vi "Simple Capture Manager.vi"() -> ()   [LabVIEW 2016]
uses:
  Simple Capture Manager Controls/Simple Capture Notifier Type.ctl
  Simple Capture Manager Controls/Simple Capture Actions.ctl
  Hardware Configuration/Hardware Configuration Controls/Device Type.ctl
  Hardware Configuration/Hardware Configuration Controls/Device Function.ctl
  Device Library/Cameras/Ximea/Ximea Controls/Ximea Actions.ctl
  Device Library/Cameras/Ximea/Ximea Controls/Ximea Parameters.ctl
  Device Library/Cameras/Ximea/Ximea Controls/Ximea Parameter List.ctl
  Simple Capture Manager Controls/Simple Capture Scan Tracker.ctl
  Device Library/Lasers/Laser Controls/Laser Actions.ctl
  Device Library/Lasers/Laser Controls/Laser Settings.ctl
  Device Library/Lasers/Laser Controls/Laser Parameters.ctl
  Device Library/Stages/Stages Controls/Stage Actions.ctl
  Device Library/Cameras/Ximea/Ximea Controls/Ximea Notifier Element.ctl
  Device Library/Cameras/Ximea/Ximea Controls/Ximea ROI.ctl
  <vilib>/vision/Image Controls.llb/IMAQ Image.ctl
  Device Library/Cameras/Camera Controls/Camera IMAQ Key Info.ctl
  shell32.dll
panel:
  in  "Quit":bool
  in  "Main Tab":enum32{"Acquisition"}(tab)
  in  "Sampling Time (s)":dbl min=0.0 format="%#_2f"
  in  "Gain":dbl=0.1
  in  "Soft trigger":bool
  out "Current Cycle":u32
  out "Cycle":sgl(slide) scale=0.0..1.0
  in  "No. of Cycles":u32=1 min=1
  out "Frame":u32(slide) scale=0.0..40.0
  in  "Base Save Path":path
  in  "Capture":bool
  in  "Preview":bool
  out "Z Step":sgl(slide) scale=0.0..1.0
  in  "File Name":string="Test Image"
  in  "Exposure Time (s)":dbl=0.1
  in  "No. of Frames":u32=1 min=1
  in  "No. of Z Steps":u32=1 min=1
  in  "Z Step Size (µm)":dbl min=-10.0 max=10.0
  out "Current Step":u32
  out "Current Frame":u32
  in  "Subfolder Name":string="Area"
  # "Live Preview"
  # "Capture"
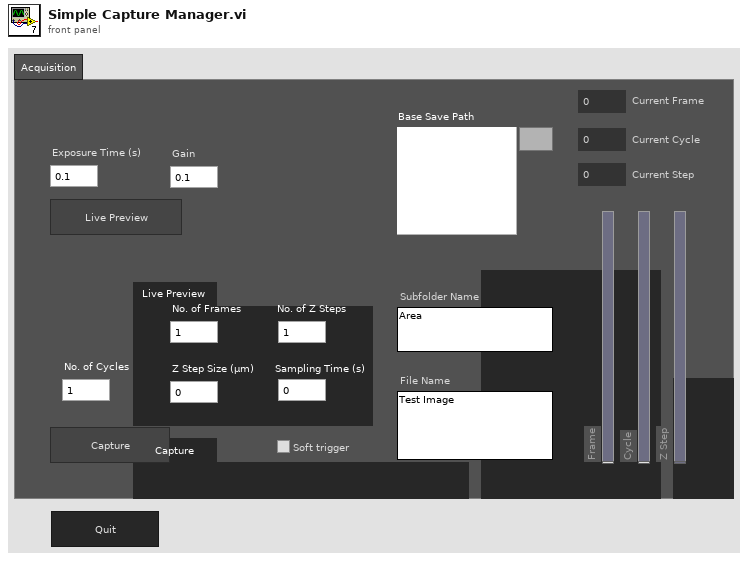
[diagram p1: front panel]
types:
  T1 = typedef "Simple Capture Notifier Type.ctl" = cluster{"No. of Frames ":u32, "No. of Z Steps":u32, "Z Step Size (µm)":dbl, "Exposure (s)":dbl, "Actions":T2, "No. of Cycles":u32, "Init Z Position (µm) ":dbl, "Base Path":path, "Save Path":path, "Metadata File Ref":refnum<file>, "Gain":dbl, "Running?":bool, "Sampling Time (s)":dbl}
  T2 = typedef "Simple Capture Actions.ctl" = enum16{"Preview", "Capture", "Laser On", "Laser Off", "Set Exposure/Gain", "Start Acquisition", "Update SubFolder", "Write Metadata", "Setup", "Camera", "Camera Soft Trigger", "Switch", "Cycle", "Step", "Abort", "Idle", "Quit"}
  T3 = typedef "Ximea Parameters.ctl" = cluster{"Parameter":T4, "Value":sgl}
  T4 = typedef "Ximea Parameter List.ctl" = enum16{"Exposure Time (s)", "Gain"}
  T5 = typedef "Device Function.ctl" = enum16{"Primary", "Secondary", "Overview", "Wide Field Drift Correction", "642 nm Excitation", "560 nm Excitation", "940 nm Excitation", "546 nm Excitation", "488 nm Excitation", "405 nm Excitation", "Objective Drift Correction", "4Pi Focus Lock", "4Pi Objective Lock", "Objective XY", "Objective Z", "Sample XY", "Sample Coarse Z", "Sample Z", "4Pi Lower", "4Pi Upper", "Mojo", "Adj Cavity", "Line Scanning", "Alert"}
  T6 = typedef "Device Type.ctl" = enum16{"AOTF", "Camera", "Deformable Mirror", "Laser", "Shutter", "Stage", "Waveform", "FPGA", "Email"}
  T7 = typedef "Ximea Actions.ctl" = enum16{"Idle", "Error Check", "Preview", "Record", "Soft Trigger", "Abort", "Record Settings", "Set Parameter", "Get Parameter", "Set ROI", "Get ROI", "Status", "Quit"}
  T8 = typedef "Simple Capture Scan Tracker.ctl" = cluster{"Current Step":u32, "Current Cycle":u32, "# of Cycles":u32, "# of Steps":u32}
  T9 = typedef "Laser Parameters.ctl" = enum16{"Wavelength (nm)", "Pulsing?", "Rep. Rate", "External Control", "Enable Fine", "Fine A", "Fine B", "Channel No."}
  T10 = typedef "Laser Settings.ctl" = cluster{"Laser Parameters":T9, "Value":dbl}
  T11 = typedef "Laser Actions.ctl" = enum16{"Error Check", "Set On/Off", "Set Power", "Set Parameter", "Get Power", "Get Status", "Get Parameter", "Quit"}
  T12 = typedef "Stage Actions.ctl" = enum16{"Get Position", "MVR", "MOVE", "HALT", "ONTARGET", "ERROR", "REFERENCE", "INIT", "VELOCITY", "STATUS", "EXIT", "HOME", "ZEROPOS", "NANOPOS", "ANALOG", "QUIT"}
  T13 = enum16{"open", "replace", "create", "open or create", "replace or create", "replace or create with confirmation"}
  T14 = typedef "Ximea Notifier Element.ctl" = cluster{"Ximea Actions":T7, "Received?":bool, "Ximea Parameter":T3, "Ximea ROI":T15, "Running?":bool, "File Path":path, "# of frames":u32, "Image Ref":T16, "Error":errorcluster, "Trigger?":bool, "ROI Increment":i32}
  T15 = typedef "Ximea ROI.ctl" = cluster{"H Offset":i32, "V Offset":i32, "H Width":i32, "V Width":i32}
  T16 = typedef "IMAQ Image.ctl" = refnum<image>
  T17 = typedef "Camera IMAQ Key Info.ctl" = cluster{"Frame":u32, "Sensor Height":i32, "Sensor Width":i32, "ROI Height":i32, "ROI Width":i32, "ROI Enable?":bool, "Bit per Pixel":u8}
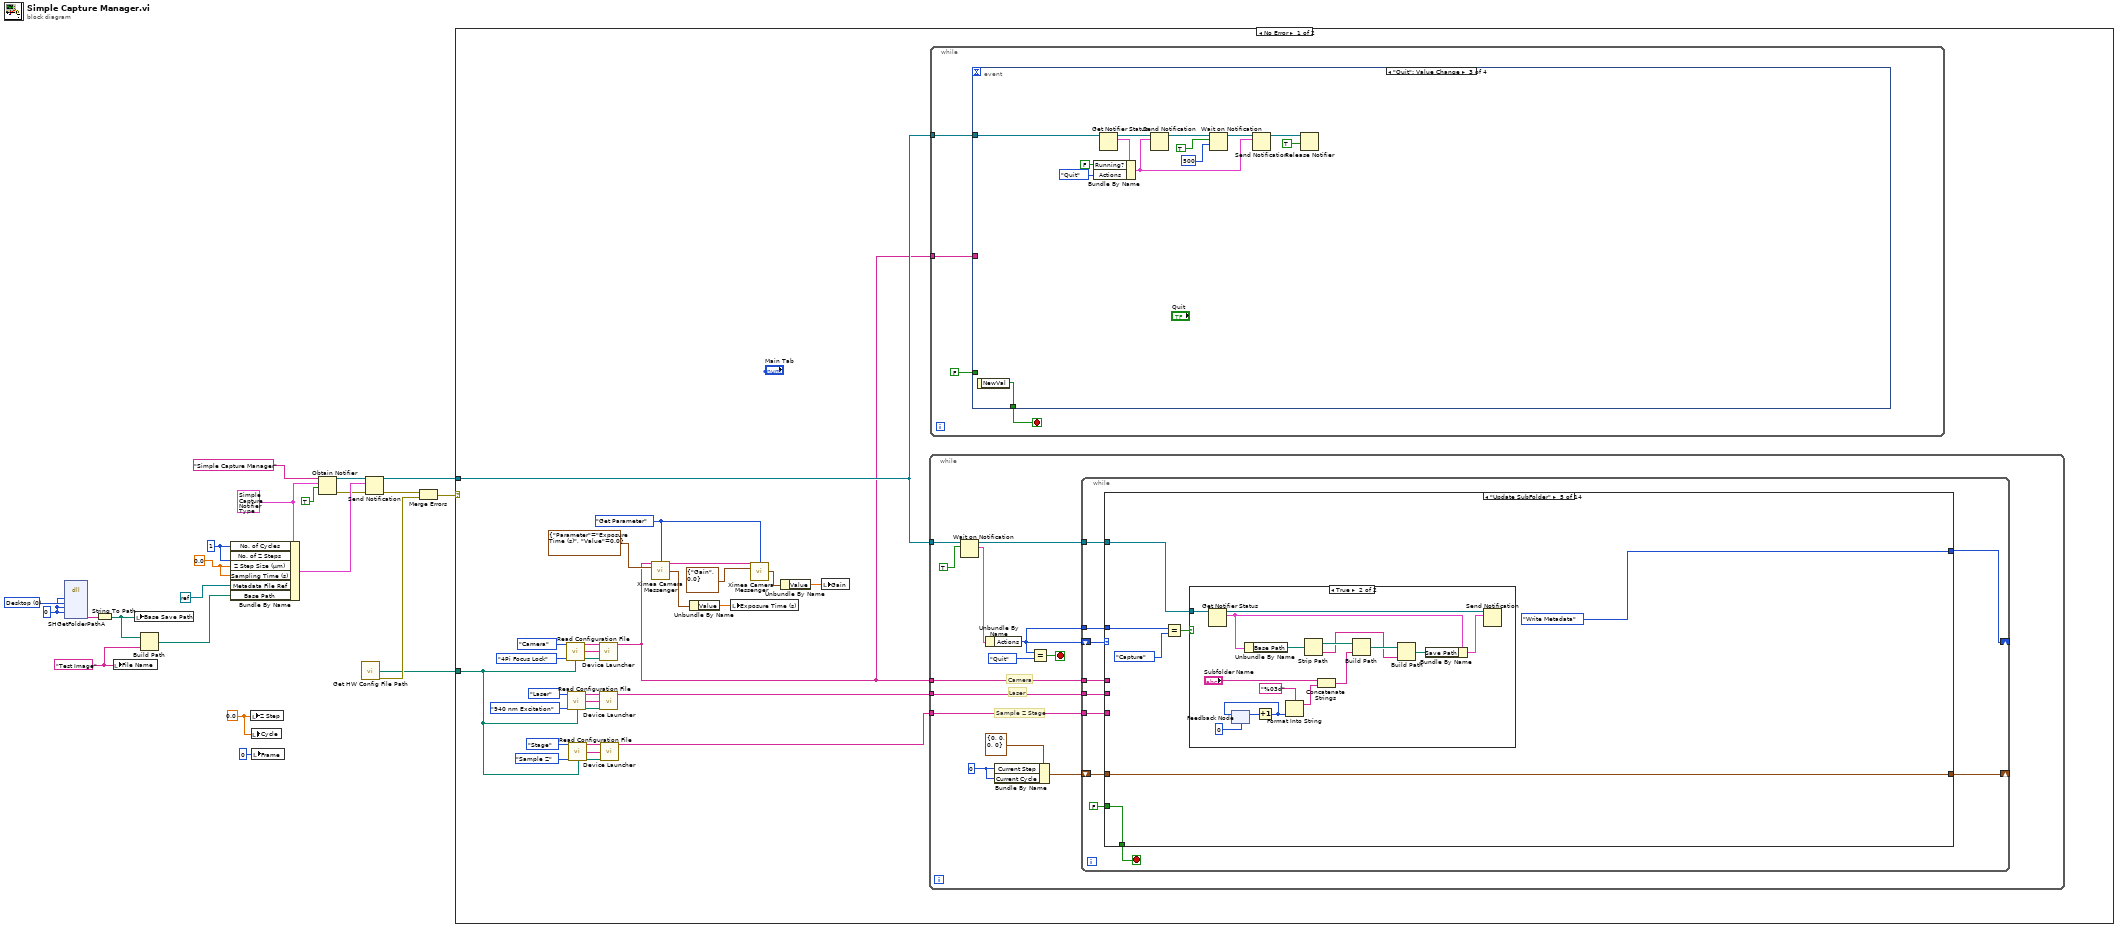
[diagram p0: block diagram]
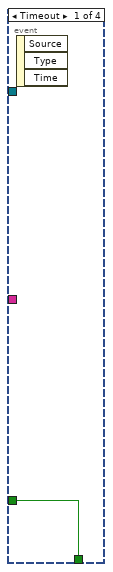
[diagram p2: hidden frame]
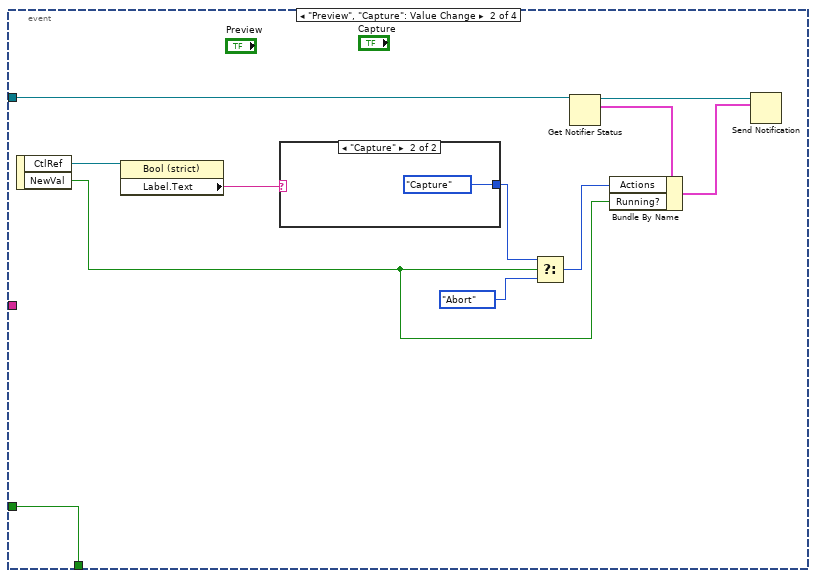
[diagram p3: hidden frame]
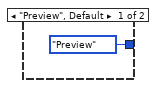
[diagram p4: hidden frame]
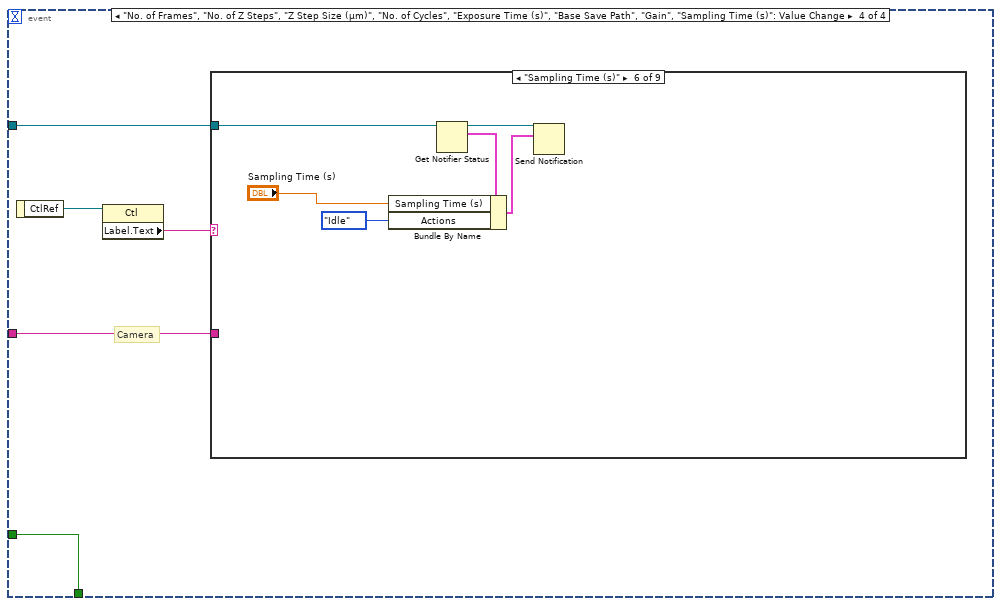
[diagram p5: hidden frame]
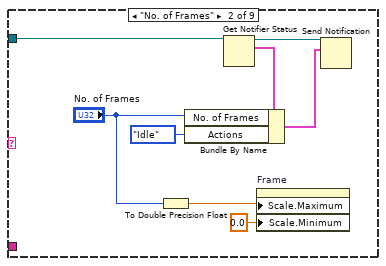
[diagram p7: hidden frame]
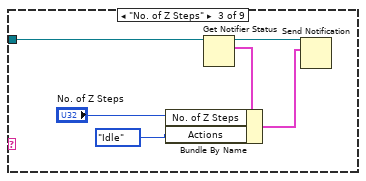
[diagram p8: hidden frame]
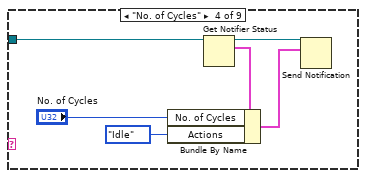
[diagram p9: hidden frame]
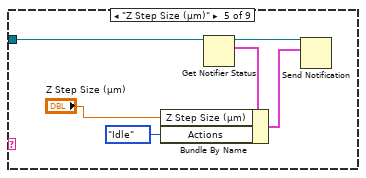
[diagram p10: hidden frame]
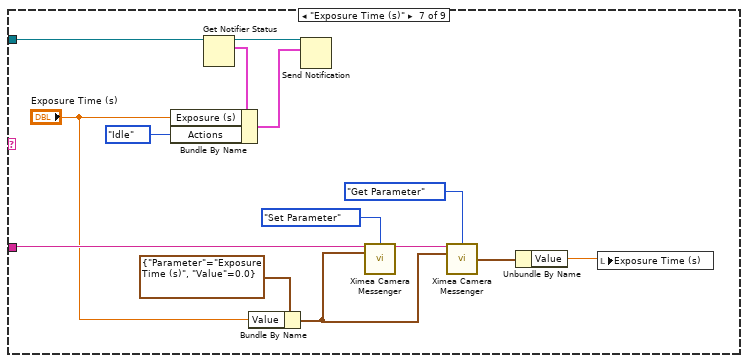
[diagram p11: hidden frame]
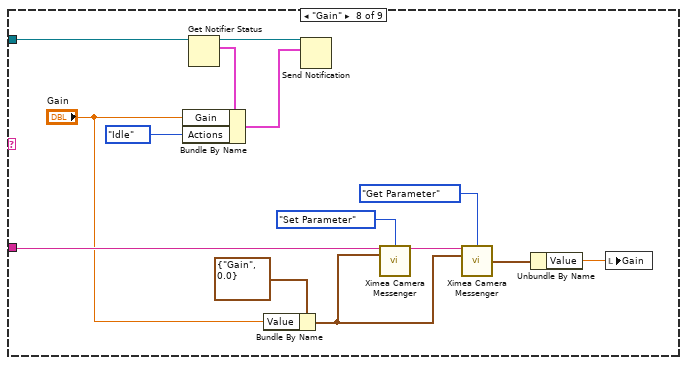
[diagram p12: hidden frame]
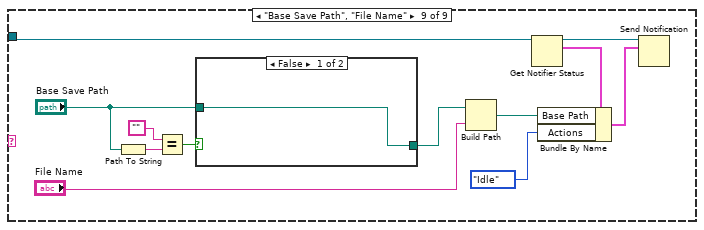
[diagram p13: hidden frame]
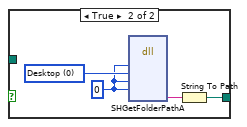
[diagram p14: hidden frame]
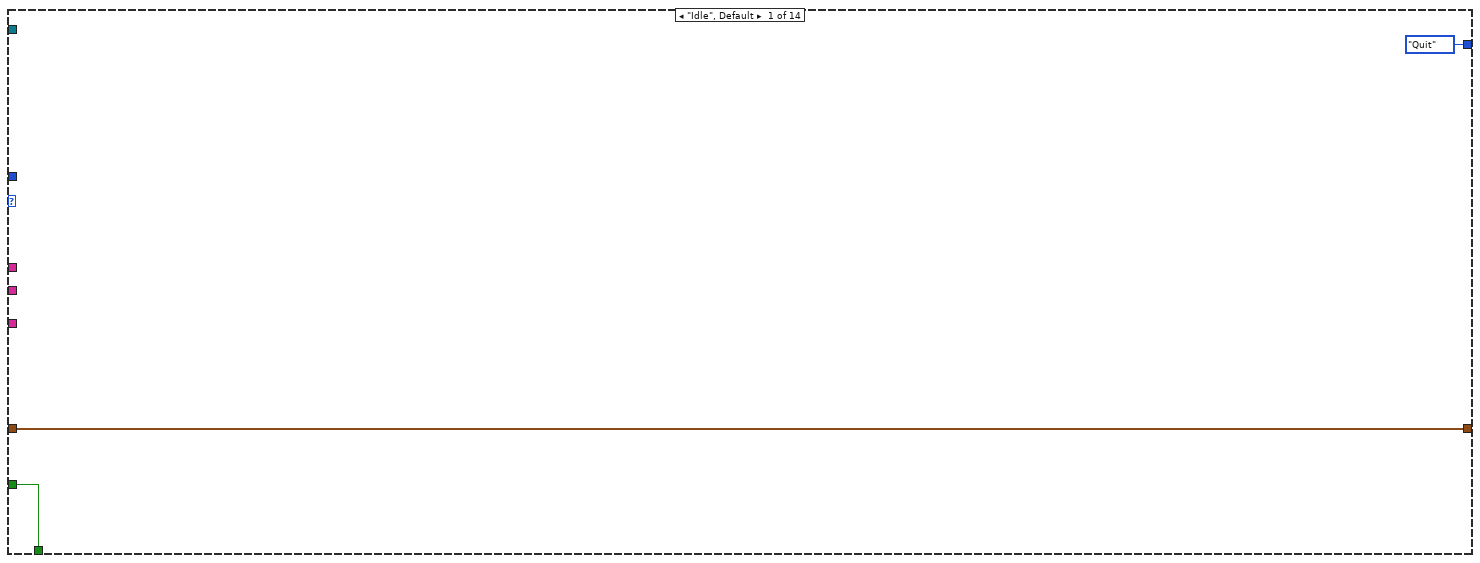
[diagram p15: hidden frame]
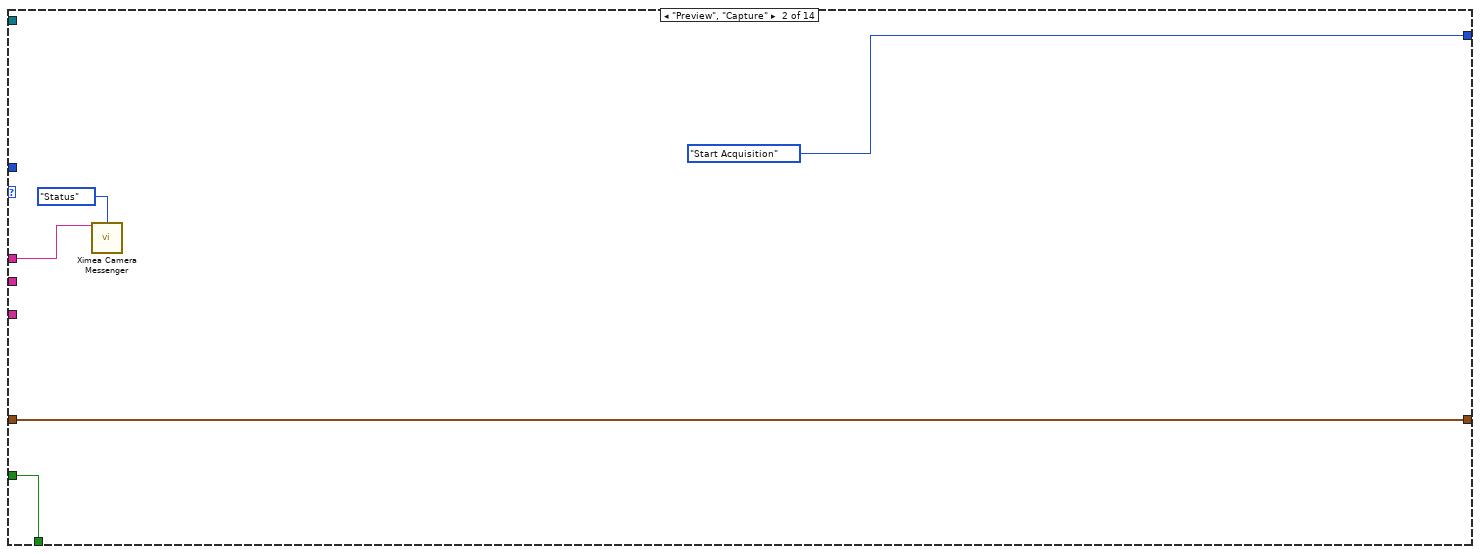
[diagram p16: hidden frame]
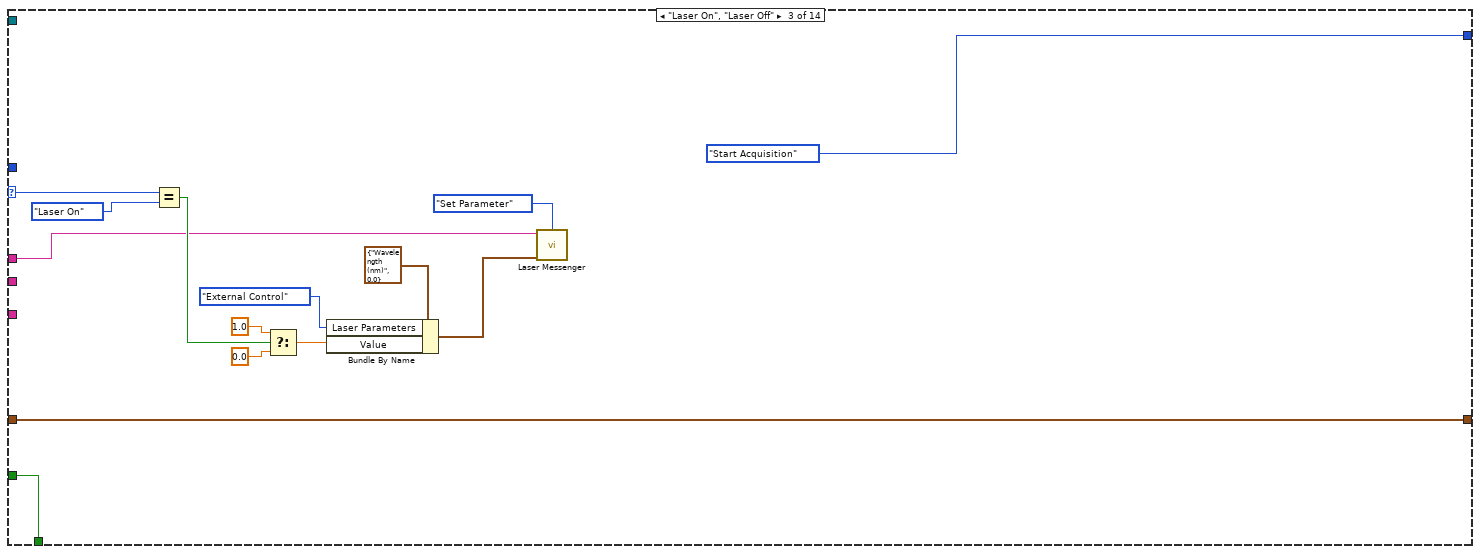
[diagram p17: hidden frame]
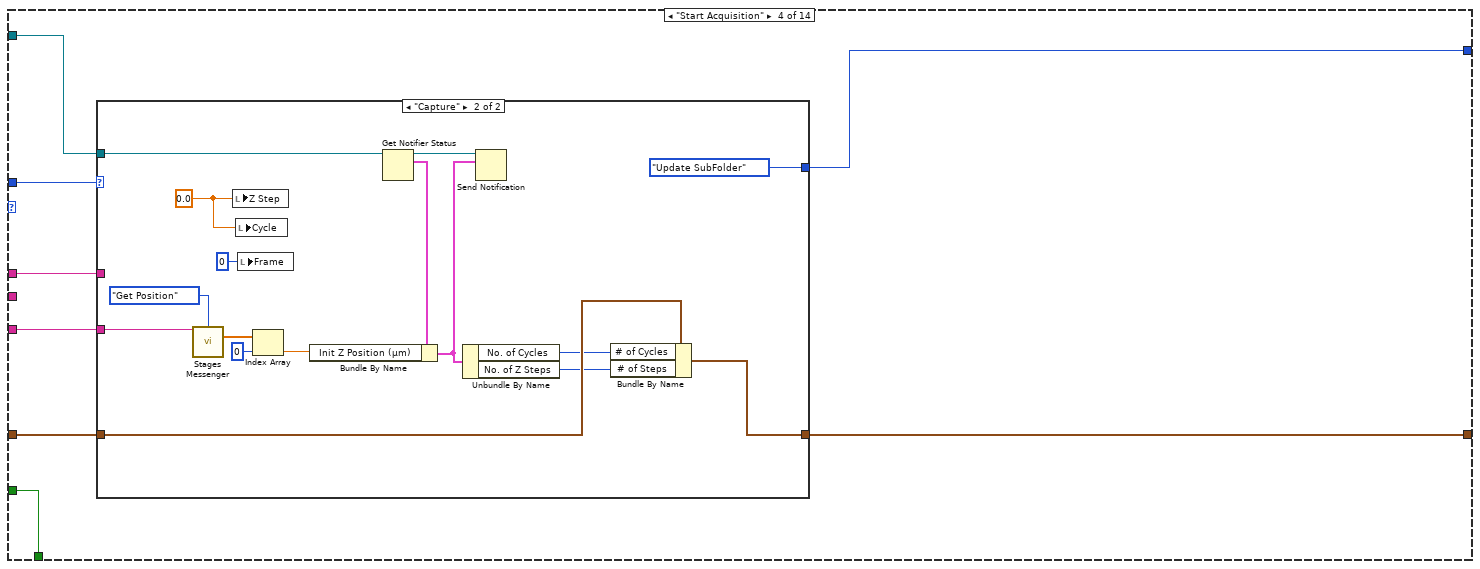
[diagram p18: hidden frame]
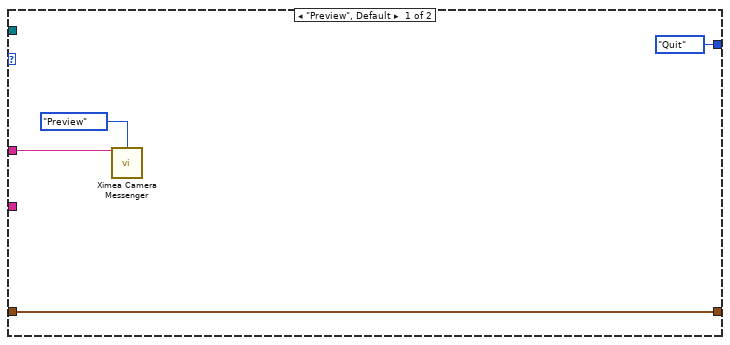
[diagram p19: hidden frame]
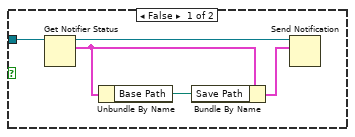
[diagram p20: hidden frame]
diagram:
  w3 = "Test Image" ("File Name")
  w7 = 0 items=["Desktop"=0, "Personal Documents"=5, "AppData"=26, "Local AppData"=28, "Common AppData"=35, "Program Files"=38, "Program Files Common"=43, "Common Documents"=46] ("Requested Path")
  w6 = 0 ("HWND")
  w9 = sgl 0.0 ("Z Step")
  w16 = u32 1 ("Cycles")
  w1 = 0.0 ("Z Step Size (µm)")
  w20 = T1 {"No. of Frames "=1, "No. of Z Steps"=1, "Z Step Size (µm)"=1.0, "Exposure (s)"=1.0, "Actions"=enum."Preview", "No. of Cycles"=1, "Init Z Position (µm) "=1.0, "Base Path"=path "", "Save Path"=path "", "Metadata File Ref"=refnum, "Gain"=1.0, "Running?"=FALSE, "Sampling Time (s)"=1.0} ("Simple Capture Notifier Type")
  n1 = dll-call lib="shell32.dll" fn="SHGetFolderPathA"("HWND"=w6, "nFolder"=w7, "hToken"=w6, "dwFlags"=w6) -> ("pszPath"=w5:string)  [unwired: 9 in, 2 out]
  n2 = String To Path(string=w5) -> (path=w4:path)
  n3 = local write "File Name"(w3) -> ()
  n4 = local write "Base Save Path"(w4) -> ()
  n5 = Build Path(base path=w4, name or relative path=w3) -> (appended path=w2:path)
  n6 = Bundle By Name(cluster=w20, "No. of Cycles"=w16, "No. of Z Steps"=w16, "Z Step Size (µm)"=w1, "Sampling Time (s)"=w1, "Metadata File Ref"=refnum<k0> refnum, "Base Path"=w2) -> (w19:T1)
  n7 = local write "Z Step"(w9) -> ()
  n8 = local write "Cycle"(w9) -> ()
  n9 = local write "Frame"(u32 0 ("Frame")) -> ()
  n10 = Obtain Notifier(name (unnamed)="Simple Capture Manager", notification data type=w20, create if not found? (T)=TRUE) -> (notifier out=w22:refnum<notifier>, error out=w18:errorcluster)  [unwired: 1 in, 1 out]
  n11 = call "Get HW Config File Path.vi"() -> ("File Path"=w11:path, "Error"=w13:errorcluster)  [unwired: 14 in]
  n12 = Send Notification(notification=w19, notifier=w22, error in (no error)=w18) -> (notifier out=w10:refnum<notifier>, error out=w14:errorcluster)
  n13 = Merge Errors(w14, w13) -> (w12:errorcluster)
  n14 = case shown="No Error" w12 {
    tunnel: w11 -> [w35 _]
    tunnel: w10 -> [w32 _]
    frame No Error {
      w28 = Ximea_Actions."Get Parameter" ("Ximea Actions")
      n15 = call "Read Configuration File.vi"("Device Type"=Device_Type."Camera", "Device Function"=Device_Function."4Pi Focus Lock", "Config File Path"=w35) -> ("Unique Notifier Name"=w50:string, "Device Ports/IDs/Channels"=w49:string[], "Device Engine Path"=w48:path)  [unwired: 9 in, 1 out]
      n16 = call "Read Configuration File.vi"("Device Type"=Device_Type."Laser", "Device Function"=Device_Function."940 nm Excitation", "Config File Path"=w35) -> ("Unique Notifier Name"=w38:string, "Device Ports/IDs/Channels"=w37:string[], "Device Engine Path"=w36:path)  [unwired: 9 in, 1 out]
      n17 = call "Read Configuration File.vi"("Device Type"=Device_Type."Stage", "Device Function"=Device_Function."Sample Z", "Config File Path"=w35) -> ("Unique Notifier Name"=w45:string, "Device Ports/IDs/Channels"=w43:string[], "Device Engine Path"=w42:path)  [unwired: 9 in, 1 out]
      n18 = call "Device Launcher.vi"("Notifier Name"=w50, "Device Ports/IDs/Channels"=w49, "Device Engine Path"=w48) -> ("Notifier Name"=w23:string)  [unwired: 11 in, 1 out]
      n19 = call "Device Launcher.vi"("Notifier Name"=w38, "Device Ports/IDs/Channels"=w37, "Device Engine Path"=w36) -> ("Notifier Name"=w34:string)  [unwired: 11 in, 1 out]
      n20 = call "Device Launcher.vi"("Notifier Name"=w45, "Device Ports/IDs/Channels"=w43, "Device Engine Path"=w42) -> ("Notifier Name"=w33:string)  [unwired: 11 in, 1 out]
      n21 = call "Ximea Camera Messenger.vi"("Notifier Name"=w23, "Ximea Actions"=w28, "Ximea  Parameter"=T3 {"Parameter"=enum."Exposure Time (s)", "Value"=0.0}) -> ("Notifier Name (Dup)"=w27:string, "Ximea Parameter Out"=w24:T3)  [unwired: 8 in, 3 out]
      n22 = Unbundle By Name(w24) -> ("Value"=w26:sgl)
      n23 = local write "Exposure Time (s)"(w26) -> ()
      n24 = call "Ximea Camera Messenger.vi"("Notifier Name"=w27, "Ximea Actions"=w28, "Ximea  Parameter"=T3 {"Parameter"=enum."Gain", "Value"=0.0}) -> ("Ximea Parameter Out"=w30:T3)  [unwired: 8 in, 4 out]
      n25 = Unbundle By Name(w30) -> ("Value"=w31:sgl)
      n26 = local write "Gain"(w31) -> ()
      n27 = while {
        tunnel: w23 -> [w171]
        tunnel: w34 -> [w170]
        tunnel: w33 -> [w169]
        tunnel: w32 -> [w176]
        stop <- w172 stop-if-true
        w165 = u32 0 ("Current Step")
        # "Sample Z Stage"
        # "Laser"
        # "Camera"
        n28 = Wait on Notification(notifier=w176, ignore previous (F)=TRUE) -> (notifier out=w167:refnum<notifier>, notification=w174:T1)  [unwired: 2 in, 2 out]
        n29 = Unbundle By Name(w174) -> ("Actions"=w168:T2)
        n30 = Bundle By Name(cluster=T8 {"Current Step"=0, "Current Cycle"=0, "# of Cycles"=0, "# of Steps"=0} ("Scan Tracker"), "Current Step"=w165, "Current Cycle"=w165) -> (w164:T8)
        n31 = Equal?(x=w168, y=Simple_Capture_Actions."Quit") -> (x = y?=w172:bool)
        n32 = while {
          tunnel: w171 -> [w186]
          shift-right: [w179] -> _
          shift-left: w168 -> [w187]
          tunnel: w170 -> [w185]
          tunnel: w169 -> [w184]
          tunnel: w168 -> [w183]
          tunnel: w167 -> [w182]
          shift-right: [w180] -> _
          shift-left: w164 -> [w181]
          stop <- w178 stop-if-true
          n33 = case shown="\"Update SubFolder\"" w187 {
            selector: w187 -> [_ _ w209 _ _ _ _ _ _ _ _ _ _ _]
            tunnel: w186 -> [_ w195 w196 w211 _ _ _ w322 w395 _ _ _ w502 _]
            tunnel: [Simple_Capture_Actions."Quit" ("f") Simple_Capture_Actions."Start Acquisition" ("Actions") Simple_Capture_Actions."Start Acquisition" ("Actions") w212 Simple_Capture_Actions."Write Metadata" ("Actions") Simple_Capture_Actions."Setup" ("Actions") w306 w315 w391 w429 w467 Simple_Capture_Actions."Setup" ("f") Simple_Capture_Actions."Quit" ("f") Simple_Capture_Actions."Quit" ("f")] -> w179
            tunnel: w185 -> [_ _ _ _ _ _ _ _ _ _ _ _ _ _]
            tunnel: w184 -> [_ _ _ w217 _ _ _ w319 _ _ w475 w494 w504 _]
            tunnel: w183 -> [_ _ _ w216 w243 _ _ _ _ _ _ _ w514 _]
            tunnel: w182 -> [_ _ _ w215 w244 w285 _ w332 w405 w453 w477 w496 w512 _]
            tunnel: w181 -> [w190 w192 w198 w214 w239 w267 w305 w314 w390 w449 w472 w491 w498 w524]
            tunnel: [w190 w192 w198 w213 w239 w267 w305 w312 w390 w427 w472 w491 w498 w524] -> w180
            tunnel: [w188 w191 w197 w210 w238 w266 w304 w310 w388 w428 w466 w489 w499 TRUE ("ignore previous (F)")] -> w178
            tunnel: FALSE ("ignore previous (F)") -> [w188 w191 w197 w210 w238 w266 w304 w310 w388 w428 w466 w489 w499 _]
            frame "Idle", Default {
            }
            frame "Preview", "Capture" {
              n34 = call "Ximea Camera Messenger.vi"("Notifier Name"=w195, "Ximea Actions"=Ximea_Actions."Status") -> ()  [unwired: 9 in, 5 out]
            }
            frame "Laser On", "Laser Off" {
              n35 = Equal?(x=w209, y=Simple_Capture_Actions."Laser On") -> (x = y?=w201:bool)
              n36 = Select(t=1.0, s=w201, f=0.0) -> (s? t:f=w203:dbl)
              n37 = Bundle By Name(cluster=T10 {"Laser Parameters"=enum."Wavelength (nm)", "Value"=0.0} ("Settings"), "Laser Parameters"=Laser_Parameters."External Control", "Value"=w203) -> (w200:T10)
              n38 = call "Laser Messenger.vi"("Notifier Name"=w196, "Action"=Laser_Actions."Set Parameter", "Laser Settings"=w200) -> ()  [unwired: 7 in, 6 out]
            }
            frame "Start Acquisition" {
              n39 = case shown="\"Capture\"" w216 {
                tunnel: w217 -> [_ w237]
                tunnel: w215 -> [_ w235]
                tunnel: w214 -> [w220 w228]
                tunnel: [w220 w225] -> w213
                tunnel: [Simple_Capture_Actions."Quit" ("Actions") Simple_Capture_Actions."Update SubFolder" ("Actions")] -> w212
                tunnel: w211 -> [w219 _]
                frame "Preview", Default {
                  n40 = call "Ximea Camera Messenger.vi"("Notifier Name"=w219, "Ximea Actions"=Ximea_Actions."Preview") -> ()  [unwired: 9 in, 5 out]
                }
                frame "Capture" {
                  w224 = sgl 0.0 ("Z Step")
                  n41 = call "Stages Messenger.vi"("Stage Notifier Name"=w237, "Actions"=Stage_Actions."Get Position") -> ("Positions"=w233:dbl[])  [unwired: 10 in, 3 out]
                  n42 = local write "Z Step"(w224) -> ()
                  n43 = local write "Cycle"(w224) -> ()
                  n44 = local write "Frame"(u32 0 ("Frame")) -> ()
                  n45 = Index Array(array=w233, index=0) -> (element=w231:dbl)
                  n46 = Get Notifier Status(notifier=w235) -> (notifier out=w230:refnum<notifier>, current notification=w234:T1)  [unwired: 1 in, 3 out]
                  n47 = Bundle By Name(cluster=w234, "Init Z Position (µm)"=w231) -> (w229:T1)
                  n48 = Unbundle By Name(w229) -> ("No. of Cycles"=w227:u32, "No. of Z Steps"=w226:u32)
                  n49 = Send Notification(notification=w229, notifier=w230) -> ()  [unwired: 1 in, 2 out]
                  n50 = Bundle By Name(cluster=w228, "# of Cycles"=w227, "# of Steps"=w226) -> (w225:T8)
                }
              }
            }
            frame "Update SubFolder" {
              n51 = Equal?(x=w243, y=Simple_Capture_Actions."Capture") -> (x = y?=w241:bool)
              n52 = case shown="True" w241 {
                tunnel: w244 -> [w249 w265]
                frame False {
                  n53 = Get Notifier Status(notifier=w249) -> (notifier out=w248:refnum<notifier>, current notification=w246:T1)  [unwired: 1 in, 3 out]
                  n54 = Unbundle By Name(w246) -> ("Base Path"=w245:path)
                  n55 = Bundle By Name(cluster=w246, "Save Path"=w245) -> (w247:T1)
                  n56 = Send Notification(notification=w247, notifier=w248) -> ()  [unwired: 1 in, 2 out]
                }
                frame True {
                  n57 = Get Notifier Status(notifier=w265) -> (notifier out=w254:refnum<notifier>, current notification=w253:T1)  [unwired: 1 in, 3 out]
                  n58 = feedback #1(u32 0) -> (w256:u32)
                  n59 = Unbundle By Name(w253) -> ("Base Path"=w264:path)
                  n60 = Increment(x=w256) -> (x+1=w255:u32)
                  n61 = feedback-in #1(w255) -> ()
                  n62 = Format Into String(format string="%03d", w255) -> (resulting string=w257:string)  [unwired: 2 in, 1 out]
                  n63 = Strip Path(path=w264) -> (stripped path=w263:path, name=w261:string)
                  n64 = Concatenate Strings("Subfolder Name", w257) -> (w260:string)
                  n65 = Build Path(base path=w263, name or relative path=w260) -> (appended path=w262:path)
                  n66 = Build Path(base path=w262, name or relative path=w261) -> (appended path=w252:path)
                  n67 = Bundle By Name(cluster=w253, "Save Path"=w252) -> (w251:T1)
                  n68 = Send Notification(notification=w251, notifier=w254) -> ()  [unwired: 1 in, 2 out]
                }
              }
            }
            frame "Write Metadata" {
              n69 = Get Notifier Status(notifier=w285) -> (notifier out=w272:refnum<notifier>, current notification=w270:T1)  [unwired: 1 in, 3 out]
              n70 = Unbundle By Name(w270) -> ("Init Z Position (µm)"=w276:dbl, "Save Path"=w275:path, "Z Step Size (µm)"=w274:dbl, "No. of Z Steps"=w273:u32)
              n71 = Less?(x=w273, y=u32 2) -> (x < y?=w282:bool)
              n72 = Equal To 0?(x=w274) -> (x = 0?=w283:bool)
              n73 = Compound Arithmetic op=OR(w283, w282) -> (w278:bool)
              n74 = Strip Path(path=w275) -> (stripped path=w279:path)  [unwired: 1 out]
              n75 = call <vilib>:"Check if File or Folder Exists.vi"("path"=w279) -> ("file or folder exists?"=w281:bool, "dup path"=w280:path)  [unwired: 8 in, 1 out]
              n76 = case shown="True" w281 {
                tunnel: [w301 w303] -> w277
                tunnel: w280 -> [w302 w303]
                frame False {
                  n77 = Create Folder(path (use dialog)=w302) -> (created path=w301:path)  [unwired: 2 in, 2 out]
                }
                frame True {
                }
              }
              n78 = case shown="False" w278 {
                tunnel: w276 -> [w297 _]
                tunnel: w277 -> [w287 _]
                tunnel: [w286 refnum<k0> refnum] -> w271
                frame False {
                  n79 = Build Path(base path=w287, name or relative path="Z Positions.txt") -> (appended path=w295:path)
                  n80 = Open/Create/Replace File(file path (use dialog)=w295, operation (0:open)=T13."replace or create") -> (refnum out=w292:refnum<file>, error out=w290:errorcluster)  [unwired: 4 in, 1 out]
                  n81 = Format Value(format string="%.4f\\n", value (0)=w297) -> (output string=w291:string)  [unwired: 1 in]
                  n82 = Write to Text File(file (use dialog)=w292, text=w291, error in=w290) -> (refnum out=w288:refnum<file>, error out=w289:errorcluster)  [unwired: 1 in, 1 out]
                  n83 = case shown="No Error" w289 {
                    tunnel: w288 -> [w298 _]
                    tunnel: [w298 refnum<k0> refnum] -> w286
                    frame No Error {
                    }
                    frame Error {
                    }
                  }
                }
                frame True {
                }
              }
              n84 = Bundle By Name(cluster=w270, "Metadata File Ref"=w271) -> (w269:T1)
              n85 = Send Notification(notification=w269, notifier=w272) -> ()  [unwired: 1 in, 2 out]
            }
            frame "Setup" {
              n86 = Select(t=Simple_Capture_Actions."Camera Soft Trigger" ("Actions"), s="Soft trigger", f=Simple_Capture_Actions."Camera") -> (s? t:f=w306:T2)
            }
            frame "Camera Soft Trigger" {
              n87 = Get Notifier Status(notifier=w332) -> (notifier out=w321:refnum<notifier>, current notification=w331:T1)  [unwired: 1 in, 3 out]
              n88 = Unbundle By Name(w331) -> ("Save Path"=w329:path, "No. of Frames"=w311:u32, "Z Step Size (µm)"=w318:dbl, "Metadata File Ref"=w317:refnum<file>)
              n89 = Unbundle By Name(w314) -> ("Current Cycle"=w328:u32, "Current Step"=w327:u32)
              n90 = call "Simple Capture File Name Increment.vi"("Path In"=w329, "Laser Line"="940", "Cycle"=w328, "Step"=w327) -> ("Path Out"=w326:path)  [unwired: 11 in]
              n91 = call "Ximea Camera Messenger.vi"("Notifier Name"=w322, "Ximea Actions"=Ximea_Actions."Record Settings", "# of Frames"=w311, "File Save Path"=w326) -> ("Notifier Name (Dup)"=w324:string)  [unwired: 7 in, 4 out]
              n92 = call "Ximea Camera Messenger.vi"("Notifier Name"=w324, "Ximea Actions"=Ximea_Actions."Soft Trigger") -> ("Notifier Name (Dup)"=w320:string, "Image Ref"=w316:T16)  [unwired: 9 in, 3 out]
              n93 = while {
                tunnel: w321 -> [w355]
                tunnel: w320 -> [w346]
                tunnel: w311 -> [w343]
                tunnel: w319 -> [w353]
                tunnel: w318 -> [w333]
                tunnel: w317 -> [w352]
                tunnel: w316 -> [w350]
                tunnel: [w336] -> w315
                tunnel: [w334] -> w313
                i -> [w349]
                stop <- w335 stop-if-true
                n94 = To Unsigned Long Integer(number=w349) -> (unsigned 32bit integer=w345:u32)
                n95 = Get Notifier Status(notifier=w355) -> (current notification=w354:T1)  [unwired: 1 in, 4 out]
                n96 = Increment(x=w345) -> (x+1=w344:u32)
                n97 = Unbundle By Name(w354) -> ("Running?"=w342:bool)
                n98 = flat-sequence {
                  tunnel: w353 -> [w361]
                  tunnel: w333 -> [w360]
                  tunnel: w352 -> [w359]
                  tunnel: [w358] -> w351
                  tunnel: w350 -> [w358]
                  tunnel: [w357] -> w348
                  tunnel: w345 -> [w357]
                  tunnel: [w356] -> w347
                  tunnel: w346 -> [w356]
                  tunnel: w351 -> [w372]
                  tunnel: w348 -> [w371]
                  tunnel: w347 -> [w365]
                  tunnel: [w362] -> w334
                  frame #0 {
                    n99 = call "Simple Capture Move Stage.vi"("Byte Stream File in"=w359, "Z Step Size (µm)"=w360, "Notifier Name"=w361) -> ()  [unwired: 9 in]
                  }
                  frame #1 {
                    n100 = Obtain Notifier(name (unnamed)=w365, notification data type=T14 {"Ximea Actions"=enum."Error Check", "Received?"=FALSE, "Ximea Parameter"={"Parameter"=enum."Exposure Time (s)", "Value"=0.0}, "Ximea ROI"={"H Offset"=0, "V Offset"=0, "H Width"=0, "V Width"=0}, "Running?"=FALSE, "File Path"=path "", "# of frames"=0, "Image Ref"=refnum, "Error"={"status"=FALSE, "code"=0, "source"=""}, "Trigger?"=FALSE, "ROI Increment"=0} ("Ximea Camera Cluster")) -> (notifier out=w370:refnum<notifier>)  [unwired: 2 in, 2 out]
                    n101 = Get Notifier Status(notifier=w370) -> (notifier out=w369:refnum<notifier>, current notification=w368:T14)  [unwired: 1 in, 3 out]
                    n102 = Bundle By Name(cluster=w368, "Trigger?"=TRUE) -> (w366:T14)
                    n103 = Send Notification(notification=w366, notifier=w369) -> (error out=w363:errorcluster)  [unwired: 1 in, 1 out]
                    n104 = while {
                      tunnel: w372 -> [w384]
                      tunnel: w363 -> [w383]
                      tunnel: [w382] -> w362
                      tunnel: w371 -> [w380]
                      i -> [w374]
                      stop <- w373 stop-if-true
                      n105 = call "IMAQ Read Custom Data"("error in (no error)"=w383, "Key"="Image Data", "Image"=w384) -> ("Custom Data Out"=w386:string)  [unwired: 6 in, 2 out]
                      n106 = Unflatten From JSON(JSON string=w386, type and defaults=T17 {"Frame"=0, "Sensor Height"=0, "Sensor Width"=0, "ROI Height"=0, "ROI Width"=0, "ROI Enable?"=FALSE, "Bit per Pixel"=0} ("Camera IMAQ Key Info")) -> (value=w385:T17)  [unwired: 5 in, 1 out]
                      n107 = Unbundle By Name(w385) -> ("Frame"=w379:u32)
                      n108 = Wait (ms)(milliseconds to wait=u32 1) -> ()  [unwired: 1 out]
                      n109 = Greater Or Equal?(x=w374, y=1000) -> (x >= y?=w375:bool)
                      n110 = Decrement(x=w379) -> (x-1=w382:u32)
                      n111 = local write "Current Frame"(w379) -> ()
                      n112 = local write "Frame"(w379) -> ()
                      n113 = Equal?(x=w382, y=w380) -> (x = y?=w376:bool)
                      n114 = Or(x=w376, y=w375) -> (x .or. y?=w373:bool)
                    }
                  }
                }
                n115 = Greater Or Equal?(x=w344, y=w343) -> (x >= y?=w341:bool)
                n116 = Not(x=w342) -> (.not. x?=w339:bool)
                n117 = Not Or(1:w341, 2:w339) -> (0:w335:bool)
                n118 = Wait (ms)(milliseconds to wait=u32 10) -> ()  [unwired: 1 out]
                n119 = Select(t=Simple_Capture_Actions."Abort" ("f"), s=w339, f=Simple_Capture_Actions."Switch") -> (s? t:f=w336:T2)
              }
              n120 = Bundle By Name(cluster=w314, "Current Step"=w313) -> (w312:T8)
            }
            frame "Camera" {
              n121 = Get Notifier Status(notifier=w405) -> (notifier out=w394:refnum<notifier>, current notification=w404:T1)  [unwired: 1 in, 3 out]
              n122 = Unbundle By Name(w390) -> ("Current Cycle"=w401:u32, "Current Step"=w400:u32)
              n123 = Unbundle By Name(w404) -> ("Save Path"=w402:path, "No. of Frames"=w389:u32)
              n124 = call "Simple Capture File Name Increment.vi"("Path In"=w402, "Laser Line"="940", "Cycle"=w401, "Step"=w400) -> ("Path Out"=w399:path)  [unwired: 11 in]
              n125 = call "Ximea Camera Messenger.vi"("Notifier Name"=w395, "Ximea Actions"=Ximea_Actions."Record Settings", "# of Frames"=w389, "File Save Path"=w399) -> ("Notifier Name (Dup)"=w397:string)  [unwired: 7 in, 4 out]
              n126 = call "Ximea Camera Messenger.vi"("Notifier Name"=w397, "Ximea Actions"=Ximea_Actions."Record") -> ("Notifier Name (Dup)"=w393:string, "Image Ref"=w392:T16)  [unwired: 9 in, 3 out]
              n127 = while {
                tunnel: w394 -> [w426]
                tunnel: w393 -> [w415]
                tunnel: w392 -> [w416]
                tunnel: [w422] -> w391
                stop <- w421 stop-if-true
                n128 = Get Notifier Status(notifier=w426) -> (current notification=w411:T1)  [unwired: 1 in, 4 out]
                n129 = Unbundle By Name(w411) -> ("Running?"=w410:bool)
                n130 = call "IMAQ Read Custom Data"("Key"="Image Data", "Image"=w416) -> ("Custom Data Out"=w419:string)  [unwired: 7 in, 2 out]
                n131 = Not(x=w410) -> (.not. x?=w407:bool)
                n132 = Unflatten From JSON(JSON string=w419, type and defaults=T17 {"Frame"=0, "Sensor Height"=0, "Sensor Width"=0, "ROI Height"=0, "ROI Width"=0, "ROI Enable?"=FALSE, "Bit per Pixel"=0} ("Camera IMAQ Key Info")) -> (value=w418:T17)  [unwired: 5 in, 1 out]
                n133 = Unbundle By Name(w418) -> ("Frame"=→"Current Frame" →"Frame":u32)
                n134 = Select(t=Ximea_Actions."Status" ("Ximea Actions"), s=w410, f=Ximea_Actions."Idle") -> (s? t:f=w412:T7)
                n135 = call "Ximea Camera Messenger.vi"("Notifier Name"=w415, "Ximea Actions"=w412) -> ("Running?"=w409:bool)  [unwired: 9 in, 4 out]
                n136 = Not(x=w409) -> (.not. x?=w408:bool)
                n137 = Or(x=w407, y=w408) -> (x .or. y?=w421:bool)
                n138 = Wait (ms)(milliseconds to wait=u32 10) -> ()  [unwired: 1 out]
                n139 = Select(t=Simple_Capture_Actions."Abort" ("f"), s=w407, f=Simple_Capture_Actions."Switch") -> (s? t:f=w422:T2)
              }
            }
            frame "Switch" {
              n140 = Get Notifier Status(notifier=w453) -> (current notification=w452:T1)  [unwired: 1 in, 4 out]
              n141 = Unbundle By Name(w452) -> ("No. of Cycles"=w451:u32, "No. of Z Steps"=w450:u32)
              n142 = Bundle By Name(cluster=w449, "# of Cycles"=w451, "# of Steps"=w450) -> (w436:T8)
              n143 = Unbundle By Name(w436) -> ("Current Cycle"=w441:u32, "# of Cycles"=w442:u32, "Current Step"=w444:u32, "# of Steps"=w443:u32)
              n144 = Increment(x=w441) -> (x+1=w438:u32)
              n145 = Increment(x=w444) -> (x+1=w437:u32)
              n146 = To Single Precision Float(number=w438) -> (single precision float=w448:sgl)
              n147 = To Single Precision Float(number=w442) -> (single precision float=w447:sgl)
              n148 = To Single Precision Float(number=w437) -> (single precision float=w446:sgl)
              n149 = To Single Precision Float(number=w443) -> (single precision float=w445:sgl)
              n150 = Divide(x=w448, y=w447) -> (x/y=→"Cycle":sgl)
              n151 = Divide(x=w446, y=w445) -> (x/y=→"Z Step":sgl)
              n152 = call "Simple Capture Scan Counter.vi"("Scan Tracker"=w436) -> ("Scan Tracker Out"=w427:T8, "To cycle?"=w433:bool, "Exit?"=w435:bool)  [unwired: 8 in]
              n153 = Select(t=Simple_Capture_Actions."Cycle" ("f"), s=w433, f=Simple_Capture_Actions."Step") -> (s? t:f=w430:T2)
              n154 = Select(t=Simple_Capture_Actions."Abort" ("f"), s=w435, f=w430) -> (s? t:f=w429:T2)
              n155 = case shown="Default" w429 {
                tunnel: w438 -> [_ _ w457]
                tunnel: w437 -> [_ w455 _]
                frame Default {
                }
                frame "Step" {
                  n156 = Increment(x=w455) -> (x+1=→"Current Step":u32)
                }
                frame "Cycle" {
                  n157 = Increment(x=w457) -> (x+1=→"Current Cycle":u32)
                }
              }
            }
            frame "Cycle" {
              n158 = Get Notifier Status(notifier=w477) -> (current notification=w476:T1)  [unwired: 1 in, 4 out]
              n159 = Unbundle By Name(w476) -> ("Init Z Position (µm)"=w474:dbl, "Z Step Size (µm)"=w461:dbl, "No. of Z Steps"=w462:u32, "Sampling Time (s)"=w458:dbl)
              n160 = Equal To 0?(x=w458) -> (x = 0?=w459:bool)
              n161 = Build Array(w474) -> (w473:dbl[])
              n162 = case shown="False" w459 {
                tunnel: w458 -> [w480 _]
                frame False {
                  n163 = Multiply(x=w480, y=1000.0) -> (x*y=w478:dbl)
                  n164 = Wait (ms)(milliseconds to wait=w478) -> ()  [unwired: 1 out]
                }
                frame True {
                }
              }
              n165 = Less?(x=w462, y=u32 2) -> (x < y?=w463:bool)
              n166 = Equal To 0?(x=w461) -> (x = 0?=w464:bool)
              n167 = Compound Arithmetic op=OR(w464, w463) -> (w460:bool)
              n168 = case shown="False" w460 {
                tunnel: w475 -> [_ w488]
                tunnel: w473 -> [_ w486]
                tunnel: [errorcluster {"status"=FALSE, "code"=0, "source"=""} ("Error") w482] -> w471
                frame True {
                }
                frame False {
                  n169 = Wait (ms)(milliseconds to wait=u32 20) -> ()  [unwired: 1 out]
                  n170 = call "Stages Messenger.vi"("Stage Notifier Name"=w488, "Actions"=Stage_Actions."MOVE", "Setpoint"=w486, "Axis"=bool[] [TRUE], "Exit While Busy?"=FALSE) -> ("Error"=w482:errorcluster)  [unwired: 7 in, 3 out]
                }
              }
              n171 = Unbundle By Name(w471) -> ("status"=w470:bool)
              n172 = Select(t=Simple_Capture_Actions."Abort" ("f"), s=w470, f=Simple_Capture_Actions."Setup") -> (s? t:f=w467:T2)
            }
            frame "Step" {
              n173 = Get Notifier Status(notifier=w496) -> (current notification=w495:T1)  [unwired: 1 in, 4 out]
              n174 = Unbundle By Name(w495) -> ("Z Step Size (µm)"=w493:dbl, "Metadata File Ref"=w492:refnum<file>)
              n175 = call "Simple Capture Move Stage.vi"("Byte Stream File in"=w492, "Z Step Size (µm)"=w493, "Notifier Name"=w494) -> ()  [unwired: 9 in]
            }
            frame "Abort" {
              n176 = call "Ximea Camera Messenger.vi"("Notifier Name"=w502, "Ximea Actions"=Ximea_Actions."Idle") -> ()  [unwired: 9 in, 5 out]
              n177 = Equal?(x=Simple_Capture_Actions."Capture", y=w514) -> (x = y?=w505:bool)
              n178 = Get Notifier Status(notifier=w512) -> (notifier out=w511:refnum<notifier>, current notification=w510:T1)  [unwired: 1 in, 3 out]
              n179 = Bundle By Name(cluster=w510, "Running?"=FALSE) -> (w508:T1)
              n180 = Unbundle By Name(w508) -> ("Metadata File Ref"=w506:refnum<file>, "Init Z Position (µm)"=w503:dbl)
              n181 = Send Notification(notification=w508, notifier=w511) -> ()  [unwired: 1 in, 2 out]
              n182 = Not A Number/Path/Refnum?(number/path/refnum=w506) -> (NaN/Path/Refnum?=w507:bool)
              n183 = case shown="False" w507 {
                tunnel: w506 -> [w521 _]
                frame False {
                  n184 = Close File(refnum=w521) -> ()  [unwired: 1 in, 2 out]
                }
                frame True {
                }
              }
              n185 = case shown="True" w505 {
                tunnel: w504 -> [_ w515]
                tunnel: w503 -> [_ w517]
                frame False {
                }
                frame True {
                  n186 = Build Array(w517) -> (w516:dbl[])
                  n187 = call "Stages Messenger.vi"("Stage Notifier Name"=w515, "Actions"=Stage_Actions."MOVE", "Setpoint"=w516, "Axis"=bool[] [TRUE], "Exit While Busy?"=FALSE) -> ()  [unwired: 7 in, 4 out]
                }
              }
              n188 = local write "Capture"(FALSE ("Capture")) -> ()
            }
            frame "Quit" {
            }
          }
        }
      }
      n189 = while {
        tunnel: w32 -> [w54]
        tunnel: w23 -> [w51]
        stop <- w53 stop-if-true
        n190 = event shown="[2] \"Quit\": Value Change" {
          selector: _ -> [_ _ _ _]
          dyn-events: _ -> [_ _ _ _]
          timeout: _ -> [_ _ _ _]
          tunnel: w54 -> [_ w64 w71 w85]
          tunnel: [w55 w58 w70 w83] -> w53
          tunnel: FALSE ("NewVal") -> [w55 w58 _ w83]
          tunnel: w51 -> [_ _ _ w82]
          event Timeout {
            n191 = event-data() -> ()  [unwired: 1 in, 3 out]
          }
          event "Preview", "Capture": Value Change {
            n192 = event-data() -> ("CtlRef"=w66:refnum<vi>, "NewVal"=w59:bool)  [unwired: 1 in]
            n193 = property class="Bool (strict)"(reference=w66) -> ("Label.Text"=w65:string)  [unwired: 1 in, 2 out]
            n194 = case shown="\"Capture\"" w65 {
              tunnel: [Simple_Capture_Actions."Preview" ("Actions") Simple_Capture_Actions."Capture" ("Actions")] -> w62
              frame "Preview", Default {
              }
              frame "Capture" {
              }
            }
            n195 = Select(t=w62, s=w59, f=Simple_Capture_Actions."Abort") -> (s? t:f=w60:T2)
            n196 = Get Notifier Status(notifier=w64) -> (notifier out=w56:refnum<notifier>, current notification=w63:T1)  [unwired: 1 in, 3 out]
            n197 = Bundle By Name(cluster=w63, "Actions"=w60, "Running?"=w59) -> (w57:T1)
            n198 = Send Notification(notification=w57, notifier=w56) -> ()  [unwired: 1 in, 2 out]
          }
          event "Quit": Value Change {
            n199 = event-data() -> ("NewVal"=w70:bool)  [unwired: 1 in]
            n200 = Get Notifier Status(notifier=w71) -> (notifier out=w81:refnum<notifier>, current notification=w80:T1)  [unwired: 1 in, 3 out]
            n201 = Bundle By Name(cluster=w80, "Running?"=FALSE ("Abort"), "Actions"=Simple_Capture_Actions."Quit") -> (w74:T1)
            n202 = Send Notification(notification=w74, notifier=w81) -> (notifier out=w78:refnum<notifier>)  [unwired: 1 in, 1 out]
            n203 = Wait on Notification(notifier=w78, ignore previous (F)=TRUE, timeout in ms (-1)=500) -> (notifier out=w75:refnum<notifier>)  [unwired: 1 in, 3 out]
            n204 = Send Notification(notification=w74, notifier=w75) -> (notifier out=w73:refnum<notifier>)  [unwired: 1 in, 1 out]
            n205 = Release Notifier(notifier=w73, force destroy? (F)=TRUE) -> ()  [unwired: 1 in, 3 out]
          }
          event "No. of Frames", "No. of Z Steps", "Z Step Size (µm)", "No. of Cycles", "Exposure Time (s)", "Base Save Path", "Gain", "Sampling Time (s)": Value Change {
            # "Camera"
            n206 = event-data() -> ("CtlRef"=w86:refnum<vi>)  [unwired: 1 in]
            n207 = property class="Ctl"(reference=w86) -> ("Label.Text"=w84:string)  [unwired: 1 in, 2 out]
            n208 = case shown="\"Sampling Time (s)\"" w84 {
              tunnel: w85 -> [_ w94 w97 w103 w109 w115 w129 w143 w150]
              tunnel: w82 -> [_ _ _ _ _ _ w126 w140 _]
              frame Default {
              }
              frame "No. of Frames" {
                n209 = To Double Precision Float(number="No. of Frames") -> (double precision float=w88:dbl)
                n210 = Get Notifier Status(notifier=w94) -> (notifier out=w91:refnum<notifier>, current notification=w93:T1)  [unwired: 1 in, 3 out]
                n211 = Bundle By Name(cluster=w93, "No. of Frames"="No. of Frames", "Actions"=Simple_Capture_Actions."Idle") -> (w92:T1)
                n212 = property on="Frame" class="Slide (strict)"("Scale.Maximum"=w88, "Scale.Minimum"=0.0 ("Scale.Range:Minimum")) -> ()  [unwired: 2 in, 2 out]
                n213 = Send Notification(notification=w92, notifier=w91) -> ()  [unwired: 1 in, 2 out]
              }
              frame "No. of Z Steps" {
                n214 = Get Notifier Status(notifier=w97) -> (notifier out=w100:refnum<notifier>, current notification=w98:T1)  [unwired: 1 in, 3 out]
                n215 = Bundle By Name(cluster=w98, "No. of Z Steps"="No. of Z Steps", "Actions"=Simple_Capture_Actions."Idle") -> (w99:T1)
                n216 = Send Notification(notification=w99, notifier=w100) -> ()  [unwired: 1 in, 2 out]
              }
              frame "No. of Cycles" {
                n217 = Get Notifier Status(notifier=w103) -> (notifier out=w106:refnum<notifier>, current notification=w104:T1)  [unwired: 1 in, 3 out]
                n218 = Bundle By Name(cluster=w104, "No. of Cycles"="No. of Cycles", "Actions"=Simple_Capture_Actions."Idle") -> (w105:T1)
                n219 = Send Notification(notification=w105, notifier=w106) -> ()  [unwired: 1 in, 2 out]
              }
              frame "Z Step Size (µm)" {
                n220 = Get Notifier Status(notifier=w109) -> (notifier out=w112:refnum<notifier>, current notification=w110:T1)  [unwired: 1 in, 3 out]
                n221 = Bundle By Name(cluster=w110, "Z Step Size (µm)"="Z Step Size (µm)", "Actions"=Simple_Capture_Actions."Idle") -> (w111:T1)
                n222 = Send Notification(notification=w111, notifier=w112) -> ()  [unwired: 1 in, 2 out]
              }
              frame "Sampling Time (s)" {
                n223 = Get Notifier Status(notifier=w115) -> (notifier out=w118:refnum<notifier>, current notification=w116:T1)  [unwired: 1 in, 3 out]
                n224 = Bundle By Name(cluster=w116, "Sampling Time (s)"="Sampling Time (s)", "Actions"=Simple_Capture_Actions."Idle") -> (w117:T1)
                n225 = Send Notification(notification=w117, notifier=w118) -> ()  [unwired: 1 in, 2 out]
              }
              frame "Exposure Time (s)" {
                n226 = Get Notifier Status(notifier=w129) -> (notifier out=w132:refnum<notifier>, current notification=w130:T1)  [unwired: 1 in, 3 out]
                n227 = Bundle By Name(cluster=w130, "Exposure (s)"="Exposure Time (s)", "Actions"=Simple_Capture_Actions."Idle") -> (w131:T1)
                n228 = Bundle By Name(cluster=T3 {"Parameter"=enum."Exposure Time (s)", "Value"=0.0} ("Ximea  Parameter"), "Value"="Exposure Time (s)") -> (w121:T3)
                n229 = Send Notification(notification=w131, notifier=w132) -> ()  [unwired: 1 in, 2 out]
                n230 = call "Ximea Camera Messenger.vi"("Notifier Name"=w126, "Ximea Actions"=Ximea_Actions."Set Parameter", "Ximea  Parameter"=w121) -> ("Notifier Name (Dup)"=w123:string)  [unwired: 8 in, 4 out]
                n231 = call "Ximea Camera Messenger.vi"("Notifier Name"=w123, "Ximea Actions"=Ximea_Actions."Get Parameter", "Ximea  Parameter"=w121) -> ("Ximea Parameter Out"=w120:T3)  [unwired: 8 in, 4 out]
                n232 = Unbundle By Name(w120) -> ("Value"=w119:sgl)
                n233 = local write "Exposure Time (s)"(w119) -> ()
              }
              frame "Gain" {
                n234 = Get Notifier Status(notifier=w143) -> (notifier out=w146:refnum<notifier>, current notification=w144:T1)  [unwired: 1 in, 3 out]
                n235 = Bundle By Name(cluster=w144, "Gain"="Gain", "Actions"=Simple_Capture_Actions."Idle") -> (w145:T1)
                n236 = Bundle By Name(cluster=T3 {"Parameter"=enum."Gain", "Value"=0.0} ("Ximea  Parameter"), "Value"="Gain") -> (w135:T3)
                n237 = Send Notification(notification=w145, notifier=w146) -> ()  [unwired: 1 in, 2 out]
                n238 = call "Ximea Camera Messenger.vi"("Notifier Name"=w140, "Ximea Actions"=Ximea_Actions."Set Parameter", "Ximea  Parameter"=w135) -> ("Notifier Name (Dup)"=w139:string)  [unwired: 8 in, 4 out]
                n239 = call "Ximea Camera Messenger.vi"("Notifier Name"=w139, "Ximea Actions"=Ximea_Actions."Get Parameter", "Ximea  Parameter"=w135) -> ("Ximea Parameter Out"=w137:T3)  [unwired: 8 in, 4 out]
                n240 = Unbundle By Name(w137) -> ("Value"=w134:sgl)
                n241 = local write "Gain"(w134) -> ()
              }
              frame "Base Save Path", "File Name" {
                n242 = Path To String(path="Base Save Path") -> (string=w154:string)
                n243 = Equal?(x="", y=w154) -> (x = y?=w152:bool)
                n244 = case shown="False" w152 {
                  tunnel: [w159 w160] -> w151
                  tunnel: "Base Save Path" -> [w159 _]
                  frame False {
                  }
                  frame True {
                    w163 = 0 items=["Desktop"=0, "Personal Documents"=5, "AppData"=26, "Local AppData"=28, "Common AppData"=35, "Program Files"=38, "Program Files Common"=43, "Common Documents"=46] ("Requested Path")
                    w162 = 0 ("HWND")
                    n245 = dll-call lib="shell32.dll" fn="SHGetFolderPathA"("HWND"=w162, "nFolder"=w163, "hToken"=w162, "dwFlags"=w162) -> ("pszPath"=w161:string)  [unwired: 9 in, 2 out]
                    n246 = String To Path(string=w161) -> (path=w160:path)
                  }
                }
                n247 = Build Path(base path=w151, name or relative path="File Name") -> (appended path=w155:path)
                n248 = Get Notifier Status(notifier=w150) -> (notifier out=w156:refnum<notifier>, current notification=w157:T1)  [unwired: 1 in, 3 out]
                n249 = Bundle By Name(cluster=w157, "Base Path"=w155, "Actions"=Simple_Capture_Actions."Idle") -> (w158:T1)
                n250 = Send Notification(notification=w158, notifier=w156) -> ()  [unwired: 1 in, 2 out]
              }
            }
          }
        }
      }
    }
    frame Error {
    }
  }
